vi "subvi Robot Manage ROI Listbox.vi"(1 "OverlapY":dbl, 3 "ROIListBoxIn":string[][](array[string]), 4 "ROIName":string, 5 "XYListOffset":u32, 6 "TileY":u32, 7 "TileX":u32, 8 "OverlapX":dbl, 9 "Selection":i32, 10 "Action":T1(ring)) -> (0 "ROIListBoxOut":string[][](array[string]), 2 "TotalROI":u32)   [LabVIEW 2012]
panel:
  out "ROITempArray":string[](array[string])
  # "1=Add, 2=Delete, 3=Rename"
  # "Sl No"
  # "Name"
  # "Tile (XxY)"
  # "XYOffsetPosition"
  # "OverlapX"
  # "OverlapY"
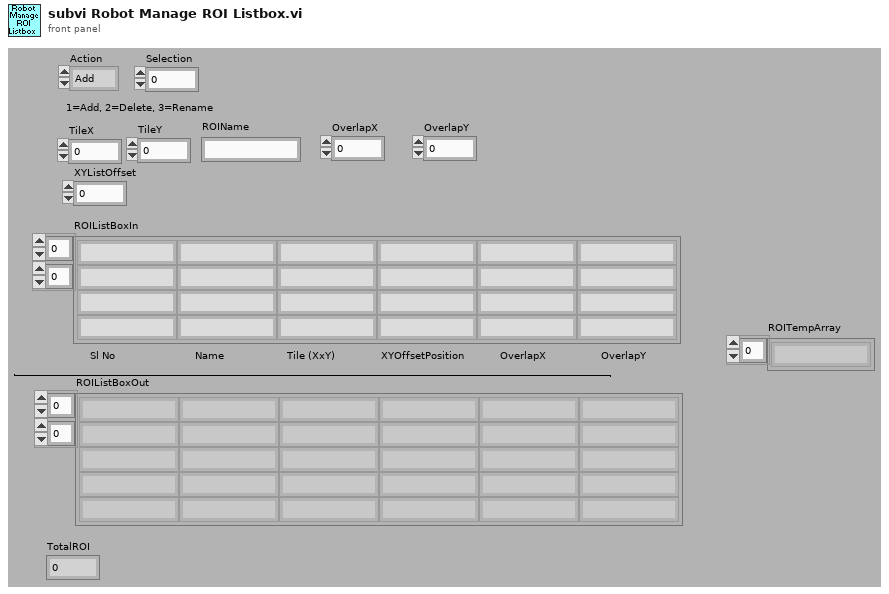
[diagram p1: front panel]
types:
  T1 = enum16{"Add", "Delete", "Rename", "Update Tiles"}
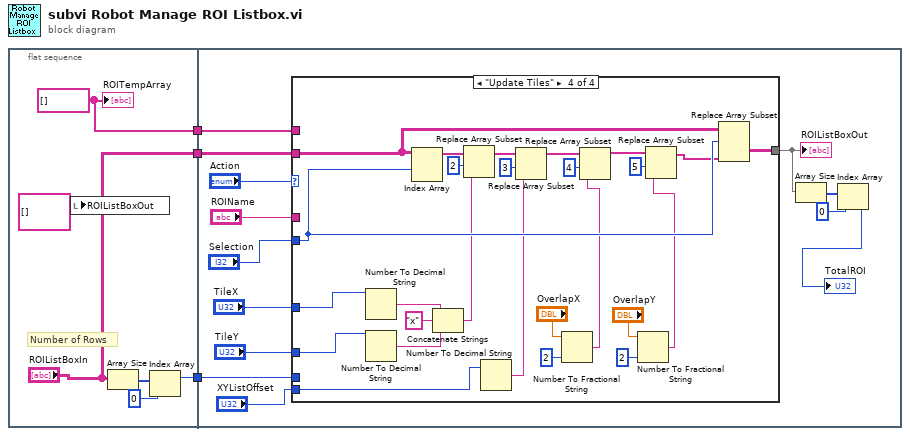
[diagram p0: block diagram]
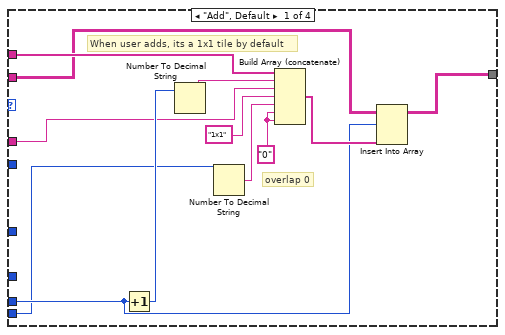
[diagram p2: hidden frame]
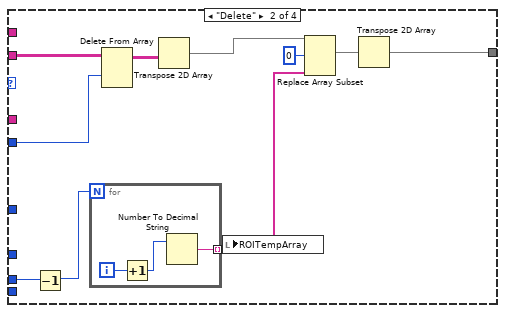
[diagram p3: hidden frame]
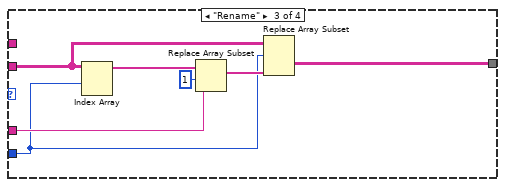
[diagram p4: hidden frame]
diagram:
  n1 = flat-sequence {
    tunnel: [w7] -> w3
    tunnel: ["ROIListBoxIn"] -> w2
    tunnel: [w5] -> w1
    tunnel: w3 -> [w21]
    tunnel: w2 -> [w20]
    tunnel: w1 -> [w19]
    frame #0 {
      w5 = string[] [] ("ROITempArray")
      # "Number of Rows"
      n2 = local write "ROIListBoxOut"(string[][] [] ("ROIListBoxOut")) -> ()
      n3 = Array Size(array="ROIListBoxIn") -> (size(s)=w9:i32[])
      n4 = Index Array(array=w9, index=0) -> (element=w7:i32)
      "ROITempArray" <- w5
    }
    frame #1 {
      n5 = case shown="\"Update Tiles\"" "Action" {
        tunnel: w21 -> [w25 w41 _ _]
        tunnel: w20 -> [w27 w44 w50 w78]
        tunnel: w19 -> [w31 _ _ _]
        tunnel: [w30 w36 w51 w70] -> w14
        tunnel: "Selection" -> [_ w35 w49 w77]
        tunnel: "ROIName" -> [w29 _ w53 _]
        tunnel: "TileX" -> [_ _ _ w73]
        tunnel: "TileY" -> [_ _ _ w72]
        tunnel: "XYListOffset" -> [w24 _ _ w66]
        frame "Add", Default {
          w23 = "0" ("string")
          # "overlap 0"
          # "When user adds, its a 1x1 tile by default"
          n6 = Increment(x=w25) -> (x+1=w34:i32)
          n7 = Number To Decimal String(number=w34) -> (decimal integer string=w32:string)  [unwired: 1 out]
          n8 = Number To Decimal String(number=w24) -> (decimal integer string=w26:string)  [unwired: 1 out]
          n9 = Build Array (concatenate)(w31, w32, w29, "1x1" ("string"), w26, w23, w23) -> (w33:string[])
          n10 = Insert Into Array(array=w27, index (row)=w25, new element=w33) -> (w30:string[][])  [unwired: 1 in]
        }
        frame "Delete" {
          n11 = Decrement(x=w41) -> (x-1=w42:i32)
          n12 = for {
            N: w42 -> [_]
            tunnel: [w45] -> w38 mode=indexing
            i -> [w47]
            n13 = Increment(x=w47) -> (x+1=w46:i32)
            n14 = Number To Decimal String(number=w46) -> (decimal integer string=w45:string)  [unwired: 1 out]
          }
          n15 = Delete From Array(array=w44, index (row)=w35) -> (array with subset deleted=w43:string[][])  [unwired: 2 in, 1 out]
          n16 = Transpose 2D Array(2D array=w43) -> (transposed array=w40:string[][])
          n17 = local write "ROITempArray"(w38) -> ()
          n18 = Replace Array Subset(array=w40, new element=w38, index (row)=0) -> (w37:string[][])  [unwired: 1 in]
          n19 = Transpose 2D Array(2D array=w37) -> (transposed array=w36:string[][])
        }
        frame "Rename" {
          n20 = Index Array(array=w50, index (row)=w49) -> (element=w48:string[])  [unwired: 1 in]
          n21 = Replace Array Subset(array=w48, new element=w53, index=1) -> (w52:string[])
          n22 = Replace Array Subset(array=w50, new element=w52, index (row)=w49) -> (w51:string[][])  [unwired: 1 in]
        }
        frame "Update Tiles" {
          n23 = Number To Decimal String(number=w73) -> (decimal integer string=w75:string)  [unwired: 1 out]
          n24 = Number To Decimal String(number=w72) -> (decimal integer string=w74:string)  [unwired: 1 out]
          n25 = Index Array(array=w78, index (row)=w77) -> (element=w79:string[])  [unwired: 1 in]
          n26 = Concatenate Strings(w75, "x" ("string"), w74) -> (w71:string)
          n27 = Replace Array Subset(array=w79, new element=w71, index=2) -> (w68:string[])
          n28 = Number To Decimal String(number=w66) -> (decimal integer string=w67:string)  [unwired: 1 out]
          n29 = Replace Array Subset(array=w68, new element=w67, index=3) -> (w63:string[])
          n30 = Number To Fractional String(number="OverlapX", precision (6)=i16 2) -> (F-format string=w57:string)  [unwired: 2 out]
          n31 = Replace Array Subset(array=w63, new element=w57, index=4) -> (w62:string[])
          n32 = Number To Fractional String(number="OverlapY", precision (6)=i16 2) -> (F-format string=w58:string)  [unwired: 2 out]
          n33 = Replace Array Subset(array=w62, new element=w58, index=5) -> (w61:string[])
          n34 = Replace Array Subset(array=w78, new element=w61, index (row)=w77) -> (w70:string[][])  [unwired: 1 in]
        }
      }
      "ROIListBoxOut" <- w14
      n35 = Array Size(array=w14) -> (size(s)=w16:i32[])
      n36 = Index Array(array=w16, index=0) -> (element=→"TotalROI":i32)
    }
  }
